vi "Actor1_GUI_G4_4.0.0_Main.vi"() -> ()   [LabVIEW 2014, in "Actor1_GUI_G4_4.0.0.lvlib"]
uses:
  <resource>/Framework/Providers/Open_GDS/ClassProviders/ActorFramework/4.0.0/Actor1_GUI_G4_4.0.0/Actor1_GUI_G4_4.0.0.lvlib
  <resource>/Framework/Providers/Open_GDS/ClassProviders/ActorFramework/4.0.0/Actor1_GUI_G4_4.0.0/Actor1_GUI_G4_4.0.0_Actor/Actor1_GUI_G4_4.0.0.lvclass
  <vilib>/ActorFramework/Message Enqueuer/Message Enqueuer.lvclass/Message Enqueuer.ctl
  <vilib>/ActorFramework/Message Enqueuer/Enqueue.vi
  <vilib>/ActorFramework/Message Priority Queue/Priority Enqueue.vi
  <vilib>/ActorFramework/Stop Msg/Stop Msg.lvclass
  <resource>/Framework/Providers/Open_GDS/ClassProviders/ActorFramework/4.0.0/Actor1_GUI_G4_4.0.0/Messages/StartMeasurement_Msg/StartMeasurement_Msg.lvclass
  <vilib>/ActorFramework/Actor/Actor.lvclass
panel:
  in  "Quit":bool
  in  "Start":bool
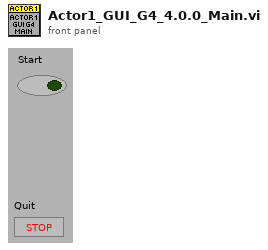
[diagram p1: front panel]
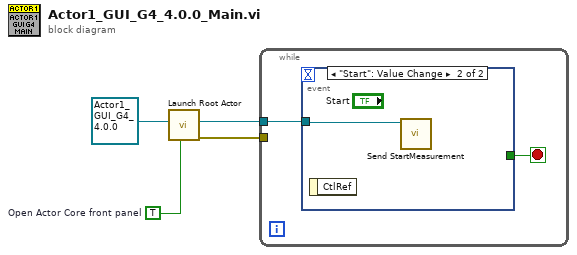
[diagram p0: block diagram]
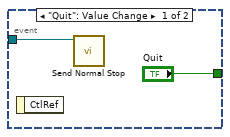
[diagram p2: hidden frame]
diagram:
  w4 = TRUE  # Open Actor Core front panel
  n1 = call <vilib>:"Launch Root Actor.vi"("Open Actor Core front panel? (F)"=w4, "Actor"=refnum<class "Actor1_GUI_G4_4.0.0.lvclass"> refnum ("Actor1_GUI_G4_4.0.0.lvlib:Actor1_GUI_G4_4.0.0")) -> ("error out"=w2:errorcluster, "Actor's Enqueuer"=w3:refnum<class "Message Enqueuer.lvclass">)  [unwired: 8 in]
  n2 = while {
    tunnel: w3 -> [w5]
    tunnel: w2 -> [_]
    stop <- w6 stop-if-true
    n3 = event shown="[1] \"Start\": Value Change" {
      selector: _ -> [_ _]
      dyn-events: _ -> [_ _]
      timeout: _ -> [_ _]
      tunnel: ["Quit" _] -> w6
      tunnel: w5 -> [w7 w9]
      event "Quit": Value Change {
        n4 = event-data() -> ()  [unwired: 1 in, 1 out]
        n5 = call <vilib>:"Send Normal Stop.vi"("Message Enqueuer"=w7) -> ()  [unwired: 10 in, 1 out]
      }
      event "Start": Value Change {
        n6 = event-data() -> ()  [unwired: 1 in, 1 out]
        n7 = call <resource>:"Send StartMeasurement.vi"("Message Enqueuer"=w9) -> ()  [unwired: 10 in, 1 out]
      }
    }
  }
